vi "ISEG_HVSystem.ProcEvents.vi"(0 "i ref in":refnum<vi>, 5 "error in (no error)":errorcluster) -> (14 "i ref out":refnum<vi>, 19 "error out":errorcluster)   [LabVIEW 2014, in "ISEG_HVSystem.lvlib"]
doc: "This method is used to define the events the object will listen to. Add your own events here."
uses:
  ISEG_HVSystem.lvlib
  CSCore/BaseProcess/BaseProcess.event definition.ctl
  CSCore/CAEObj/CAEObj.event definition.ctl
  CSCore/BaseProcess/BaseProcess.descriptor string definition.ctl
  CSCore/BaseProcess/BaseProcess.lvlib
  CSCore/CAEObj/CAEObj.lvlib
panel:
  in  "event definition":T1={"CAEEvtDef"={"URL"="lvmsg://setKill", "enable"=TRUE, "ignoreResID"=FALSE}, "Data Descriptor"="S:1 n[Kill] //If Kill=True: Switch OFF at the max rate all system channels;"}
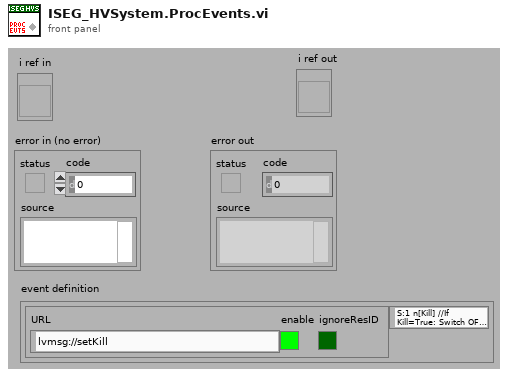
[diagram p1: front panel]
types:
  T1 = typedef "BaseProcess.lvlib/BaseProcess.event definition.ctl" = cluster{"CAEEvtDef":T2, "Data Descriptor":T3}
  T2 = typedef "CAEObj.lvlib/CAEObj.event definition.ctl" = cluster{"URL":string, "enable":bool, "ignoreResID":bool}
  T3 = typedef "BaseProcess.lvlib/BaseProcess.descriptor string definition.ctl" = string
  T4 = typedef "ISEG_HVSystem.lvlib/ISEG_HVSystem.i attribute.ctl" = cluster{"System Name":string, "CAN_Status bus":cluster{"CAN":string, "DIM Status":T5}, "Client Active?":cluster{"Active":bool, "DIM Status":T5}, "Client Connected?":cluster{"Connected":bool, "DIM Status":T5}, "OPC Version":cluster{"OPC Version":string, "DIM Status":T5}, "Pr ID":cluster{"Pr ID":string, "DIM Status":T5}, " Modell":string, " Prefix":string, "Force":cluster{"Force":bool, "DIM Status":T5}, "Refresh":cluster{"Refresh":dbl, "DIM Status":T5}}
  T5 = typedef "ISEG_HVSystem.lvlib/ISEG_HVSystem.DIM Status.ctl" = cluster{"no link":bool, "quality":i32, "Time Stamp":timestamp}
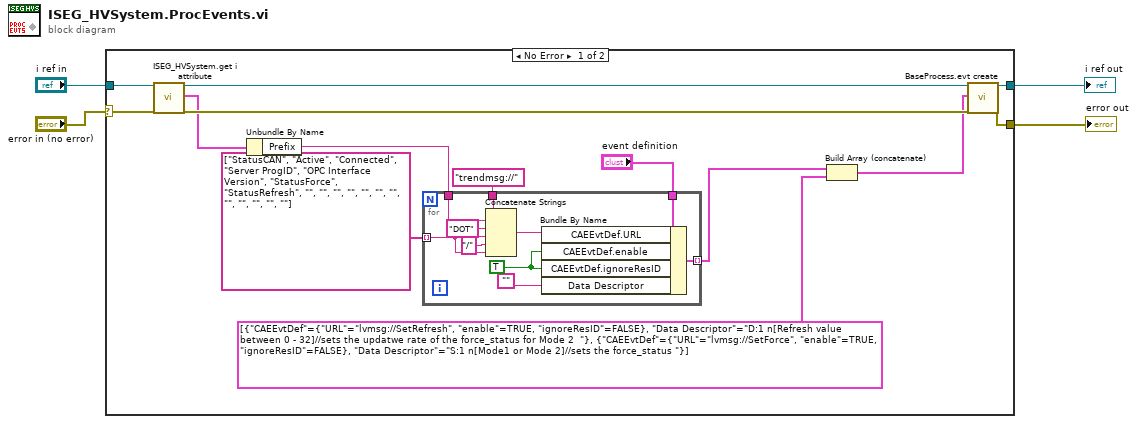
[diagram p0: block diagram]
diagram:
  n1 = case shown="No Error" "error in (no error)" {
    selector: "error in (no error)" -> [w12 w29]
    tunnel: "i ref in" -> [w13 w30]
    tunnel: [w18 w30] -> w1
    tunnel: [w17 w29] -> w2
    frame No Error {
      n2 = call "ISEG_HVSystem.get i attribute.vi"("i ref in"=w13, "error in (no error)"=w12) -> ("i ref out"=w11:refnum<vi>, "i attribute"=w9:T4, "error out"=w10:errorcluster)  [unwired: 15 in]
      n3 = Unbundle By Name(w9) -> ("Prefix"=w8:string)
      n4 = for {
        tunnel: "event definition" -> [w28]
        tunnel: "trendmsg://" -> [w27]
        tunnel: string[] ["StatusCAN", "Active", "Connected", "Server ProgID", "OPC Interface Version", "StatusForce", "StatusRefresh", "", "", "", "", "", "", "", "", "", "", "", ""] -> [w22] mode=indexing
        tunnel: [w21] -> w7 mode=indexing
        tunnel: w8 -> [w20]
        w25 = TRUE ("CAEEvtDef.ignoreResID")
        n5 = Concatenate Strings(w27, w20, "DOT" ("string"), w22, "/" ("string"), w22) -> (w26:string)
        n6 = Bundle By Name(cluster=w28, "CAEEvtDef.URL"=w26, "CAEEvtDef.enable"=w25, "CAEEvtDef.ignoreResID"=w25, "Data Descriptor"="") -> (w21:T1)
      }
      n7 = Build Array (concatenate)(w7, T1[] [{"CAEEvtDef"={"URL"="lvmsg://SetRefresh", "enable"=TRUE, "ignoreResID"=FALSE}, "Data Descriptor"="D:1 n[Refresh value between 0 - 32]//sets the updatwe rate of the force_status for Mode 2  "}, {"CAEEvtDef"={"URL"="lvmsg://SetForce", "enable"=TRUE, "ignoreResID"=FALSE}, "Data Descriptor"="S:1 n[Mode1 or Mode 2]//sets the force_status "}]) -> (w5:T1[])
      n8 = call "BaseProcess.evt create.vi"("i ref in"=w11, "newEvents"=w5, "error in (no error)"=w10) -> ("i ref out"=w18:refnum<vi>, "error out"=w17:errorcluster)  [unwired: 13 in, 2 out]
    }
    frame Error {
    }
  }
  "i ref out" <- w1
  "error out" <- w2
